vi "border.vi"(8 "Error in":errorcluster caption="Error in (no error)", 10 "Border Parameters (in)":T1, 11 "Border Radio (in)":i32) -> (0 "Error out":errorcluster, 2 "Border Parameters (out)":T1, 3 "Border Radio (out)":i32, 4 "Border Time (ms)":dbl)   [LabVIEW 2018]
uses:
  Controls/gradient_parameters.ctl
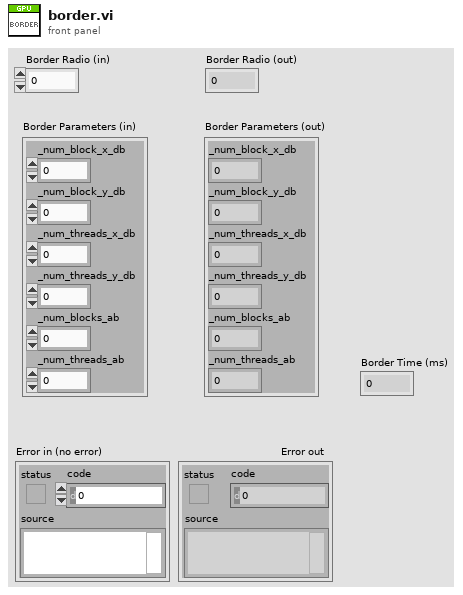
[diagram p1: front panel]
types:
  T1 = typedef "gradient_parameters.ctl" = cluster{"_num_block_x_db":i32, "_num_block_y_db":i32, "_num_threads_x_db":i32, "_num_threads_y_db":i32, "_num_blocks_ab":i32, "_num_threads_ab":i32}
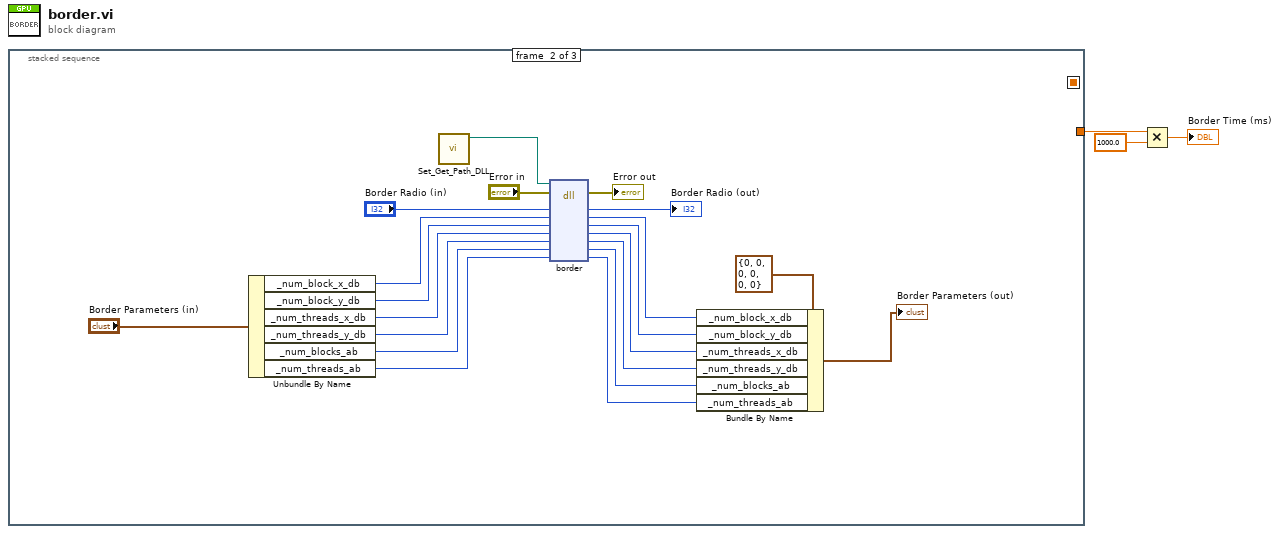
[diagram p0: block diagram]
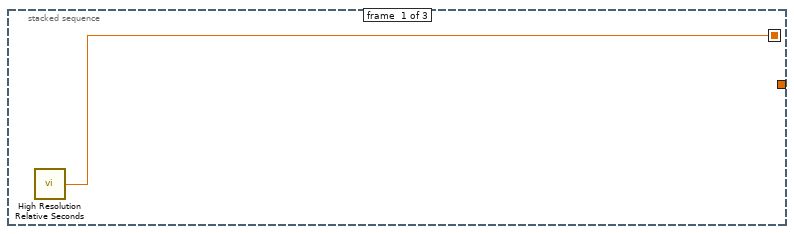
[diagram p2: hidden frame]
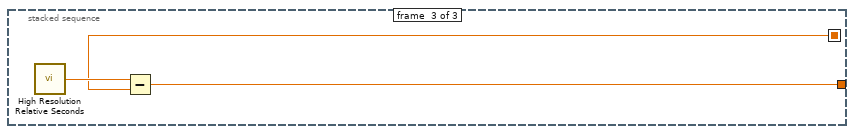
[diagram p3: hidden frame]
diagram:
  n1 = stacked-sequence {
    seq-local: [w4 _ _] -> [_ _ w26]
    tunnel: [_ _ w25] -> w1
    frame #0 {
      n2 = call <vilib>:"High Resolution Relative Seconds.vi"() -> ("relative seconds"=w4:dbl)
    }
    frame #1 {
      n3 = Unbundle By Name("Border Parameters (in)") -> ("_num_block_x_db"=w19:i32, "_num_block_y_db"=w18:i32, "_num_threads_x_db"=w17:i32, "_num_threads_y_db"=w16:i32, "_num_blocks_ab"=w15:i32, "_num_threads_ab"=w14:i32)
      n4 = call "Set_Get_Path_DLL.vi"() -> ("path DLL Out"=w5:path)  [unwired: 11 in]
      n5 = dll-call lib="C:/Users/AUTIS/Documents/TFG/Proyecto/Visual Studio/SR_GPU_TOOLKIT_INIT/x64/Release/SR_GPU_TOOLKIT.dll" fn="border"(path in=w5, error in="Error in", "radio"="Border Radio (in)", "_num_block_x_db"=w19, "_num_block_y_db"=w18, "_num_threads_x_db"=w17, "_num_threads_y_db"=w16, "_num_blocks_ab"=w15, "_num_threads_ab"=w14) -> (error out=→"Error out":errorcluster, "radio"=→"Border Radio (out)":i32, "_num_block_x_db"=w11:i32, "_num_block_y_db"=w10:i32, "_num_threads_x_db"=w9:i32, "_num_threads_y_db"=w8:i32, "_num_blocks_ab"=w7:i32, "_num_threads_ab"=w6:i32)  [unwired: 2 in, 1 out]
      n6 = Bundle By Name(cluster=T1 {"_num_block_x_db"=0, "_num_block_y_db"=0, "_num_threads_x_db"=0, "_num_threads_y_db"=0, "_num_blocks_ab"=0, "_num_threads_ab"=0} ("Gradient Parameters (out)"), "_num_block_x_db"=w11, "_num_block_y_db"=w10, "_num_threads_x_db"=w9, "_num_threads_y_db"=w8, "_num_blocks_ab"=w7, "_num_threads_ab"=w6) -> (→"Border Parameters (out)":T1)
    }
    frame #2 {
      n7 = call <vilib>:"High Resolution Relative Seconds.vi"() -> ("relative seconds"=w27:dbl)
      n8 = Subtract(x=w27, y=w26) -> (x-y=w25:dbl)
    }
  }
  n9 = Multiply(x=w1, y=1000.0) -> (x*y=→"Border Time (ms)":dbl)
